vi "树型.vi"() -> ()   [LabVIEW 2010]
panel:
  in  "树形":string(tree)
  out "字符串":string
  in  "树形":string(tree)
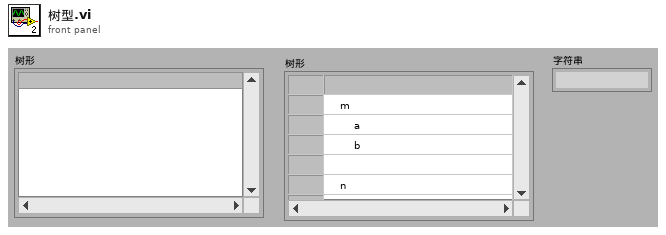
[diagram p1: front panel]
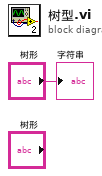
[diagram p0: block diagram]
diagram:
  "字符串" <- "树形"
